vi "instr.DSO1002A.vi"(7 "SignalVpp(V)":dbl, 8 "错误输入（无错误）":errorcluster, 9 "SignalFreq(kHz)":dbl, 10 "CMD":T1(ring), 11 "VISA资源名称":refnum<visa-resource-name>) -> (0 "错误输出":errorcluster, 2 "Return Value":dbl, 3 "OK?":bool)   [LabVIEW 2012, in "Lib_UEL.ATE.lvlib" / "Lib_Instrument.lvlib"]
uses:
  Lib_Instrument.lvlib
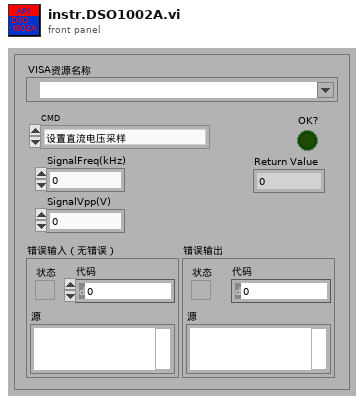
[diagram p1: front panel]
types:
  T1 = enum16{"设置直流电压采样", "获取直流电压值", "设置RMS采样", "获取RMS值", "设置频率采样", "获取频率值", "获取VPP", "重设Timing", "设置频率采用(10k LowPass)"}
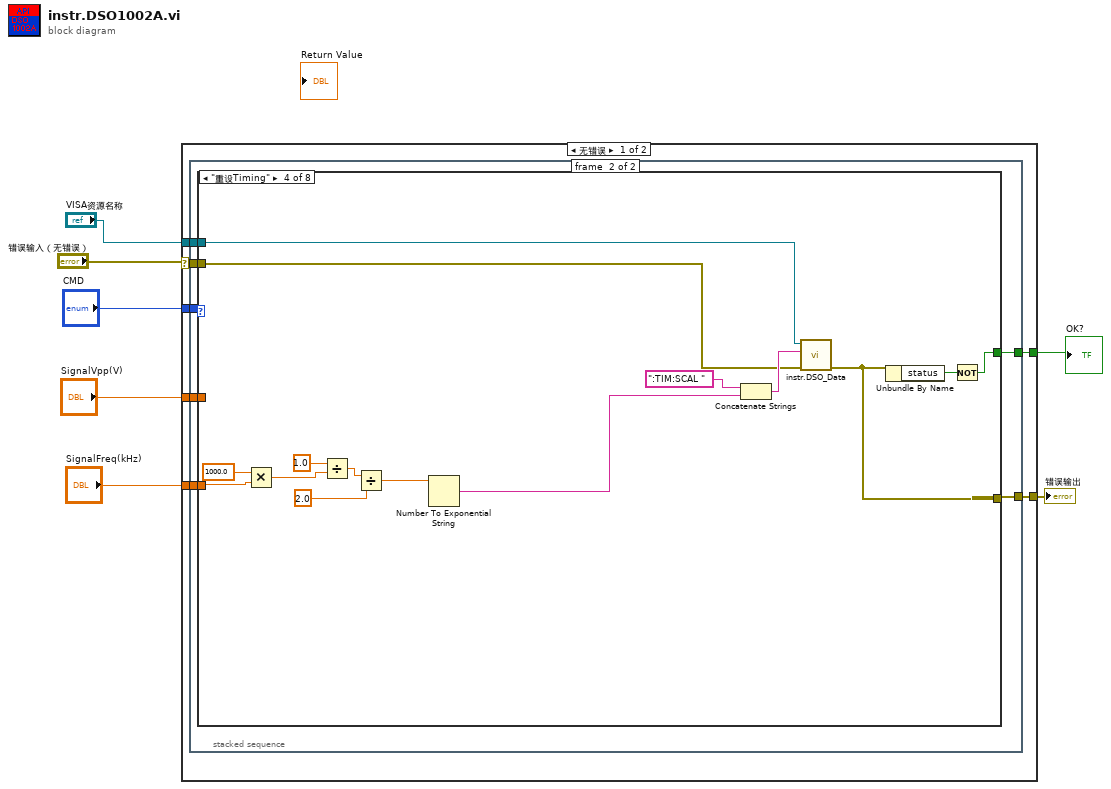
[diagram p0: block diagram]
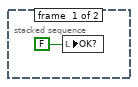
[diagram p2: hidden frame]
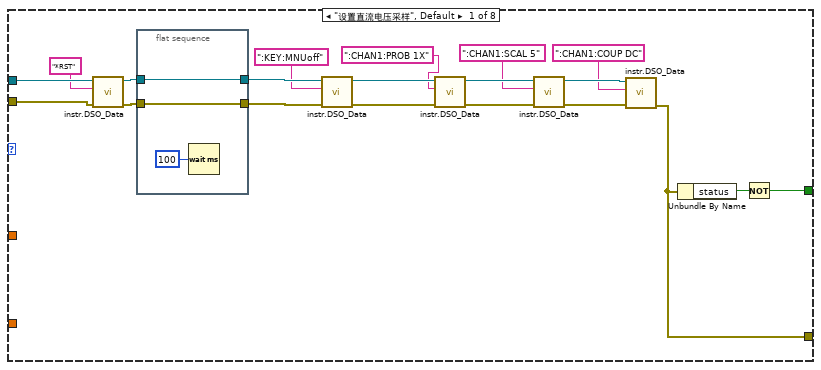
[diagram p3: hidden frame]
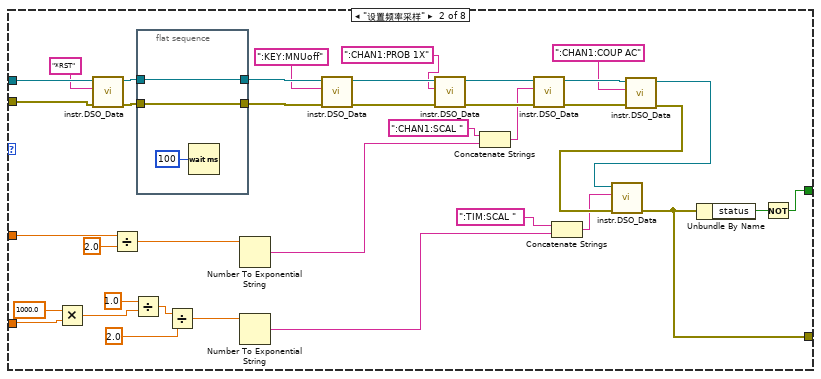
[diagram p4: hidden frame]
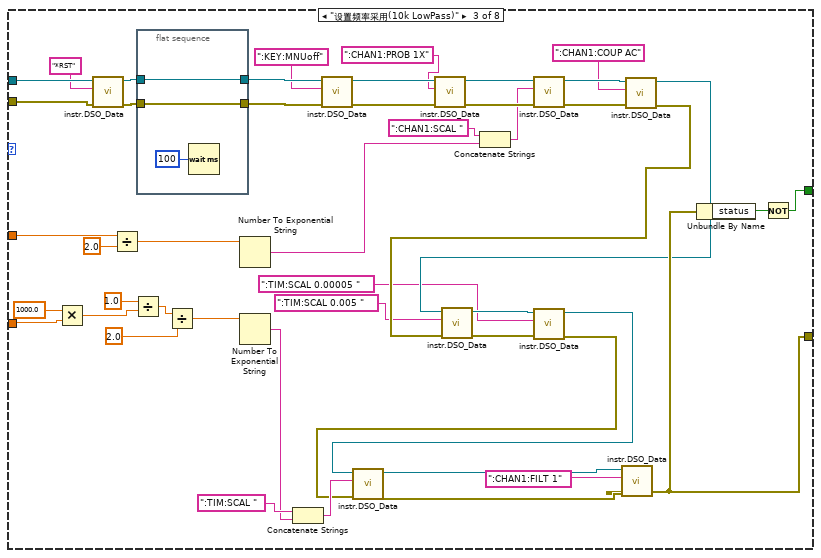
[diagram p5: hidden frame]
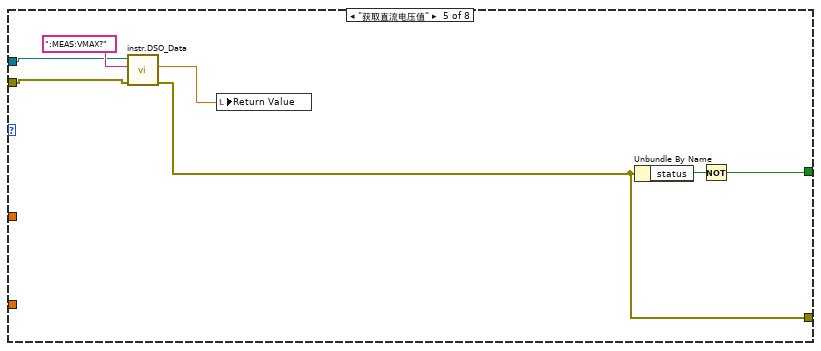
[diagram p6: hidden frame]
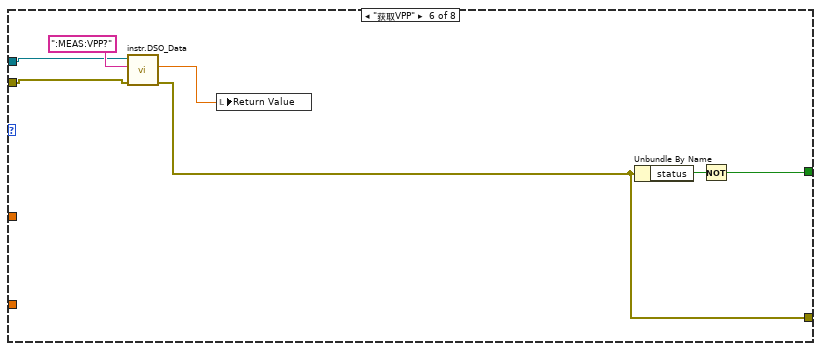
[diagram p7: hidden frame]
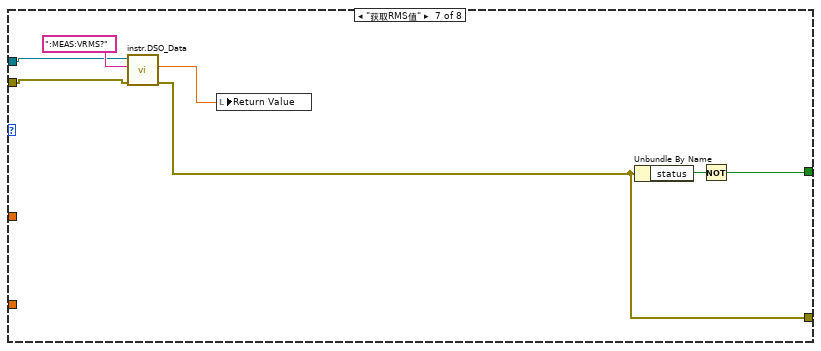
[diagram p8: hidden frame]
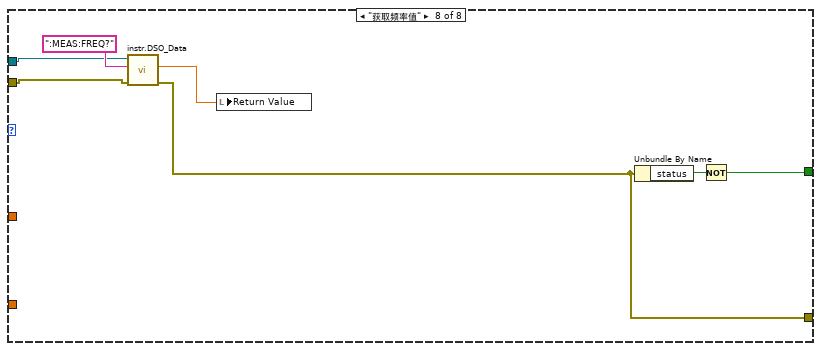
[diagram p9: hidden frame]
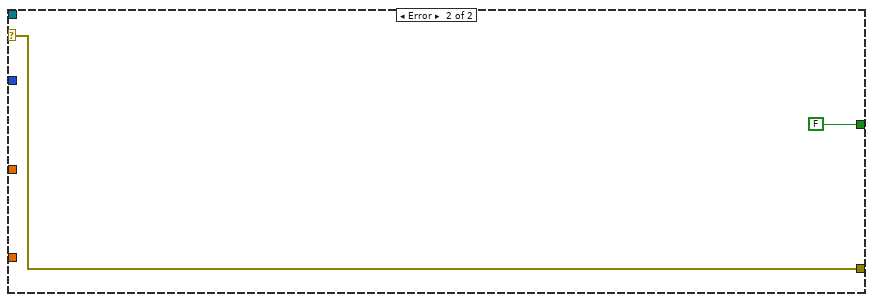
[diagram p10: hidden frame]
diagram:
  n1 = case shown="无错误" "错误输入（无错误）" {
    selector: "错误输入（无错误）" -> [w12 w179]
    tunnel: [w11 w179] -> w6
    tunnel: "VISA资源名称" -> [w14 _]
    tunnel: "CMD" -> [w13 _]
    tunnel: [w10 FALSE] -> w3
    tunnel: "SignalFreq(kHz)" -> [w9 _]
    tunnel: "SignalVpp(V)" -> [w8 _]
    frame No Error {
      n2 = stacked-sequence {
        tunnel: w14 -> [_ w22]
        tunnel: w13 -> [_ w21]
        tunnel: w12 -> [_ w20]
        tunnel: [_ w19] -> w11
        tunnel: [_ w18] -> w10
        tunnel: w9 -> [_ w17]
        tunnel: w8 -> [_ w16]
        frame #0 {
          n3 = local write "OK?"(FALSE ("OK?")) -> ()
        }
        frame #1 {
          n4 = case shown="\"重设Timing\"" w21 {
            tunnel: w22 -> [w42 w82 w131 w136 w155 w162 w169 w176]
            tunnel: w20 -> [w41 w81 w130 w135 w154 w161 w168 w175]
            tunnel: [w25 w52 w94 w137 w150 w157 w164 w171] -> w19
            tunnel: [w23 w65 w114 w148 w151 w158 w165 w172] -> w18
            tunnel: w17 -> [_ w61 w110 w144 _ _ _ _]
            tunnel: w16 -> [_ w51 w103 _ _ _ _ _]
            frame "设置直流电压采样", Default {
              n5 = call "instr.DSO_Data.vi"("错误输入（无错误）"=w41, "CMD write"="*RST", "VISA.in"=w42) -> ("错误输出"=w36:errorcluster, "VISA.out"=w38:refnum<visa-resource-name>)  [unwired: 5 in, 2 out]
              n6 = flat-sequence {
                tunnel: [w44] -> w39
                tunnel: w38 -> [w44]
                tunnel: [w43] -> w37
                tunnel: w36 -> [w43]
                frame #0 {
                  n7 = Wait (ms)(milliseconds to wait=u32 100 ("等待时间（毫秒）")) -> ()  [unwired: 1 out]
                }
              }
              n8 = call "instr.DSO_Data.vi"("错误输入（无错误）"=w37, "CMD write"=":KEY:MNUoff", "VISA.in"=w39) -> ("错误输出"=w33:errorcluster, "VISA.out"=w34:refnum<visa-resource-name>)  [unwired: 5 in, 2 out]
              n9 = call "instr.DSO_Data.vi"("错误输入（无错误）"=w33, "CMD write"=":CHAN1:PROB 1X", "VISA.in"=w34) -> ("错误输出"=w30:errorcluster, "VISA.out"=w31:refnum<visa-resource-name>)  [unwired: 5 in, 2 out]
              n10 = call "instr.DSO_Data.vi"("错误输入（无错误）"=w30, "CMD write"=":CHAN1:SCAL 5", "VISA.in"=w31) -> ("错误输出"=w27:errorcluster, "VISA.out"=w28:refnum<visa-resource-name>)  [unwired: 5 in, 2 out]
              n11 = call "instr.DSO_Data.vi"("错误输入（无错误）"=w27, "CMD write"=":CHAN1:COUP DC", "VISA.in"=w28) -> ("错误输出"=w25:errorcluster)  [unwired: 5 in, 3 out]
              n12 = Unbundle By Name(w25) -> ("status"=w24:bool)
              n13 = Not(x=w24) -> (.not. x?=w23:bool)
            }
            frame "设置频率采样" {
              n14 = Multiply(x=1000.0, y=w61) -> (x*y=w60:dbl)
              n15 = call "instr.DSO_Data.vi"("错误输入（无错误）"=w81, "CMD write"="*RST", "VISA.in"=w82) -> ("错误输出"=w76:errorcluster, "VISA.out"=w78:refnum<visa-resource-name>)  [unwired: 5 in, 2 out]
              n16 = Divide(x=w51, y=2.0) -> (x/y=w48:dbl)
              n17 = Divide(x=1.0, y=w60) -> (x/y=w63:dbl)
              n18 = flat-sequence {
                tunnel: [w84] -> w79
                tunnel: w78 -> [w84]
                tunnel: [w83] -> w77
                tunnel: w76 -> [w83]
                frame #0 {
                  n19 = Wait (ms)(milliseconds to wait=u32 100 ("等待时间（毫秒）")) -> ()  [unwired: 1 out]
                }
              }
              n20 = Divide(x=w63, y=2.0) -> (x/y=w58:dbl)
              n21 = Number To Exponential String(number=w48) -> (E-format string=w47:string)  [unwired: 3 in]
              n22 = Number To Exponential String(number=w58) -> (E-format string=w54:string)  [unwired: 3 in]
              n23 = call "instr.DSO_Data.vi"("错误输入（无错误）"=w77, "CMD write"=":KEY:MNUoff", "VISA.in"=w79) -> ("错误输出"=w73:errorcluster, "VISA.out"=w74:refnum<visa-resource-name>)  [unwired: 5 in, 2 out]
              n24 = call "instr.DSO_Data.vi"("错误输入（无错误）"=w73, "CMD write"=":CHAN1:PROB 1X", "VISA.in"=w74) -> ("错误输出"=w70:errorcluster, "VISA.out"=w71:refnum<visa-resource-name>)  [unwired: 5 in, 2 out]
              n25 = Concatenate Strings(":CHAN1:SCAL " ("CMD write"), w47) -> (w46:string)
              n26 = call "instr.DSO_Data.vi"("错误输入（无错误）"=w70, "CMD write"=w46, "VISA.in"=w71) -> ("错误输出"=w68:errorcluster, "VISA.out"=w69:refnum<visa-resource-name>)  [unwired: 5 in, 2 out]
              n27 = Concatenate Strings(":TIM:SCAL " ("CMD write"), w54) -> (w53:string)
              n28 = call "instr.DSO_Data.vi"("错误输入（无错误）"=w68, "CMD write"=":CHAN1:COUP AC", "VISA.in"=w69) -> ("错误输出"=w56:errorcluster, "VISA.out"=w57:refnum<visa-resource-name>)  [unwired: 5 in, 2 out]
              n29 = call "instr.DSO_Data.vi"("错误输入（无错误）"=w56, "CMD write"=w53, "VISA.in"=w57) -> ("错误输出"=w52:errorcluster)  [unwired: 5 in, 3 out]
              n30 = Unbundle By Name(w52) -> ("status"=w66:bool)
              n31 = Not(x=w66) -> (.not. x?=w65:bool)
            }
            frame "设置频率采用(10k LowPass)" {
              n32 = Multiply(x=1000.0, y=w110) -> (x*y=w109:dbl)
              n33 = call "instr.DSO_Data.vi"("错误输入（无错误）"=w130, "CMD write"="*RST", "VISA.in"=w131) -> ("错误输出"=w125:errorcluster, "VISA.out"=w127:refnum<visa-resource-name>)  [unwired: 5 in, 2 out]
              n34 = Divide(x=w103, y=2.0) -> (x/y=w100:dbl)
              n35 = Divide(x=1.0, y=w109) -> (x/y=w112:dbl)
              n36 = flat-sequence {
                tunnel: [w133] -> w128
                tunnel: w127 -> [w133]
                tunnel: [w132] -> w126
                tunnel: w125 -> [w132]
                frame #0 {
                  n37 = Wait (ms)(milliseconds to wait=u32 100 ("等待时间（毫秒）")) -> ()  [unwired: 1 out]
                }
              }
              n38 = Divide(x=w112, y=2.0) -> (x/y=w107:dbl)
              n39 = Number To Exponential String(number=w100) -> (E-format string=w99:string)  [unwired: 3 in]
              n40 = Number To Exponential String(number=w107) -> (E-format string=w105:string)  [unwired: 3 in]
              n41 = Concatenate Strings(":TIM:SCAL " ("CMD write"), w105) -> (w104:string)
              n42 = call "instr.DSO_Data.vi"("错误输入（无错误）"=w126, "CMD write"=":KEY:MNUoff", "VISA.in"=w128) -> ("错误输出"=w122:errorcluster, "VISA.out"=w123:refnum<visa-resource-name>)  [unwired: 5 in, 2 out]
              n43 = call "instr.DSO_Data.vi"("错误输入（无错误）"=w122, "CMD write"=":CHAN1:PROB 1X", "VISA.in"=w123) -> ("错误输出"=w119:errorcluster, "VISA.out"=w120:refnum<visa-resource-name>)  [unwired: 5 in, 2 out]
              n44 = Concatenate Strings(":CHAN1:SCAL " ("CMD write"), w99) -> (w98:string)
              n45 = call "instr.DSO_Data.vi"("错误输入（无错误）"=w119, "CMD write"=w98, "VISA.in"=w120) -> ("错误输出"=w117:errorcluster, "VISA.out"=w118:refnum<visa-resource-name>)  [unwired: 5 in, 2 out]
              n46 = call "instr.DSO_Data.vi"("错误输入（无错误）"=w117, "CMD write"=":CHAN1:COUP AC", "VISA.in"=w118) -> ("错误输出"=w88:errorcluster, "VISA.out"=w91:refnum<visa-resource-name>)  [unwired: 5 in, 2 out]
              n47 = call "instr.DSO_Data.vi"("错误输入（无错误）"=w88, "CMD write"=":TIM:SCAL 0.005 ", "VISA.in"=w91) -> ("错误输出"=w92:errorcluster, "VISA.out"=w93:refnum<visa-resource-name>)  [unwired: 5 in, 2 out]
              n48 = call "instr.DSO_Data.vi"("错误输入（无错误）"=w92, "CMD write"=":TIM:SCAL 0.00005 ", "VISA.in"=w93) -> ("错误输出"=w89:errorcluster, "VISA.out"=w90:refnum<visa-resource-name>)  [unwired: 5 in, 2 out]
              n49 = call "instr.DSO_Data.vi"("错误输入（无错误）"=w89, "CMD write"=w104, "VISA.in"=w90) -> ("错误输出"=w97:errorcluster, "VISA.out"=w96:refnum<visa-resource-name>)  [unwired: 5 in, 2 out]
              n50 = call "instr.DSO_Data.vi"("错误输入（无错误）"=w97, "CMD write"=":CHAN1:FILT 1", "VISA.in"=w96) -> ("错误输出"=w94:errorcluster)  [unwired: 5 in, 3 out]
              n51 = Unbundle By Name(w94) -> ("status"=w115:bool)
              n52 = Not(x=w115) -> (.not. x?=w114:bool)
            }
            frame "重设Timing" {
              n53 = Multiply(x=1000.0, y=w144) -> (x*y=w143:dbl)
              n54 = Divide(x=1.0, y=w143) -> (x/y=w146:dbl)
              n55 = Divide(x=w146, y=2.0) -> (x/y=w141:dbl)
              n56 = Number To Exponential String(number=w141) -> (E-format string=w139:string)  [unwired: 3 in]
              n57 = Concatenate Strings(":TIM:SCAL " ("CMD write"), w139) -> (w138:string)
              n58 = call "instr.DSO_Data.vi"("错误输入（无错误）"=w135, "CMD write"=w138, "VISA.in"=w136) -> ("错误输出"=w137:errorcluster)  [unwired: 5 in, 3 out]
              n59 = Unbundle By Name(w137) -> ("status"=w149:bool)
              n60 = Not(x=w149) -> (.not. x?=w148:bool)
            }
            frame "获取直流电压值" {
              n61 = call "instr.DSO_Data.vi"("错误输入（无错误）"=w154, "CMD write"=":MEAS:VMAX?", "VISA.in"=w155) -> ("错误输出"=w150:errorcluster, "Value"=w153:dbl)  [unwired: 5 in, 2 out]
              n62 = local write "Return Value"(w153) -> ()
              n63 = Unbundle By Name(w150) -> ("status"=w152:bool)
              n64 = Not(x=w152) -> (.not. x?=w151:bool)
            }
            frame "获取VPP" {
              n65 = call "instr.DSO_Data.vi"("错误输入（无错误）"=w161, "CMD write"=":MEAS:VPP?", "VISA.in"=w162) -> ("错误输出"=w157:errorcluster, "Value"=w160:dbl)  [unwired: 5 in, 2 out]
              n66 = local write "Return Value"(w160) -> ()
              n67 = Unbundle By Name(w157) -> ("status"=w159:bool)
              n68 = Not(x=w159) -> (.not. x?=w158:bool)
            }
            frame "获取RMS值" {
              n69 = call "instr.DSO_Data.vi"("错误输入（无错误）"=w168, "CMD write"=":MEAS:VRMS?", "VISA.in"=w169) -> ("错误输出"=w164:errorcluster, "Value"=w167:dbl)  [unwired: 5 in, 2 out]
              n70 = local write "Return Value"(w167) -> ()
              n71 = Unbundle By Name(w164) -> ("status"=w166:bool)
              n72 = Not(x=w166) -> (.not. x?=w165:bool)
            }
            frame "获取频率值" {
              n73 = call "instr.DSO_Data.vi"("错误输入（无错误）"=w175, "CMD write"=":MEAS:FREQ?", "VISA.in"=w176) -> ("错误输出"=w171:errorcluster, "Value"=w174:dbl)  [unwired: 5 in, 2 out]
              n74 = local write "Return Value"(w174) -> ()
              n75 = Unbundle By Name(w171) -> ("status"=w173:bool)
              n76 = Not(x=w173) -> (.not. x?=w172:bool)
            }
          }
        }
      }
    }
    frame Error {
    }
  }
  "错误输出" <- w6
  "OK?" <- w3
